vi "Main.vi"() -> ()   [LabVIEW 2013]
uses:
  <vilib>/myRIO/Common/Instrument Driver Framework/myRIO v1.0/UART/vis/myRIO v1.0 Close UART.vi
  <vilib>/myRIO/Common/Instrument Driver Framework/Utilities/vis/FPGA Ref Manager.vi
  <vilib>/myRIO/Common/Instrument Driver Framework/myRIO v1.0/myRIO v1.0 Reset FPGA.vi
  <vilib>/myRIO/Instrument Drivers/Utilities/Utilities.lvlib
panel:
  in  "Stop Button":bool
  out "logfile":path
  out "datalog record":T1
  # "Data Logger -- light+temp"
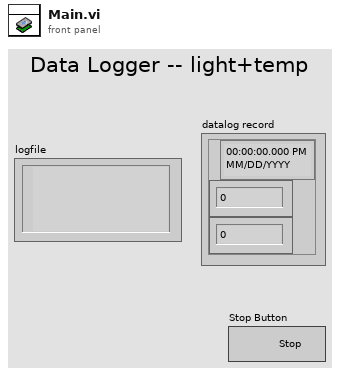
[diagram p1: front panel]
types:
  T1 = cluster{timestamp, "Numeric Control":u8, "Numeric Control":dbl}
  T2 = enum16{"open", "replace", "create", "open or create", "replace or create", "replace or create with confirmation"}
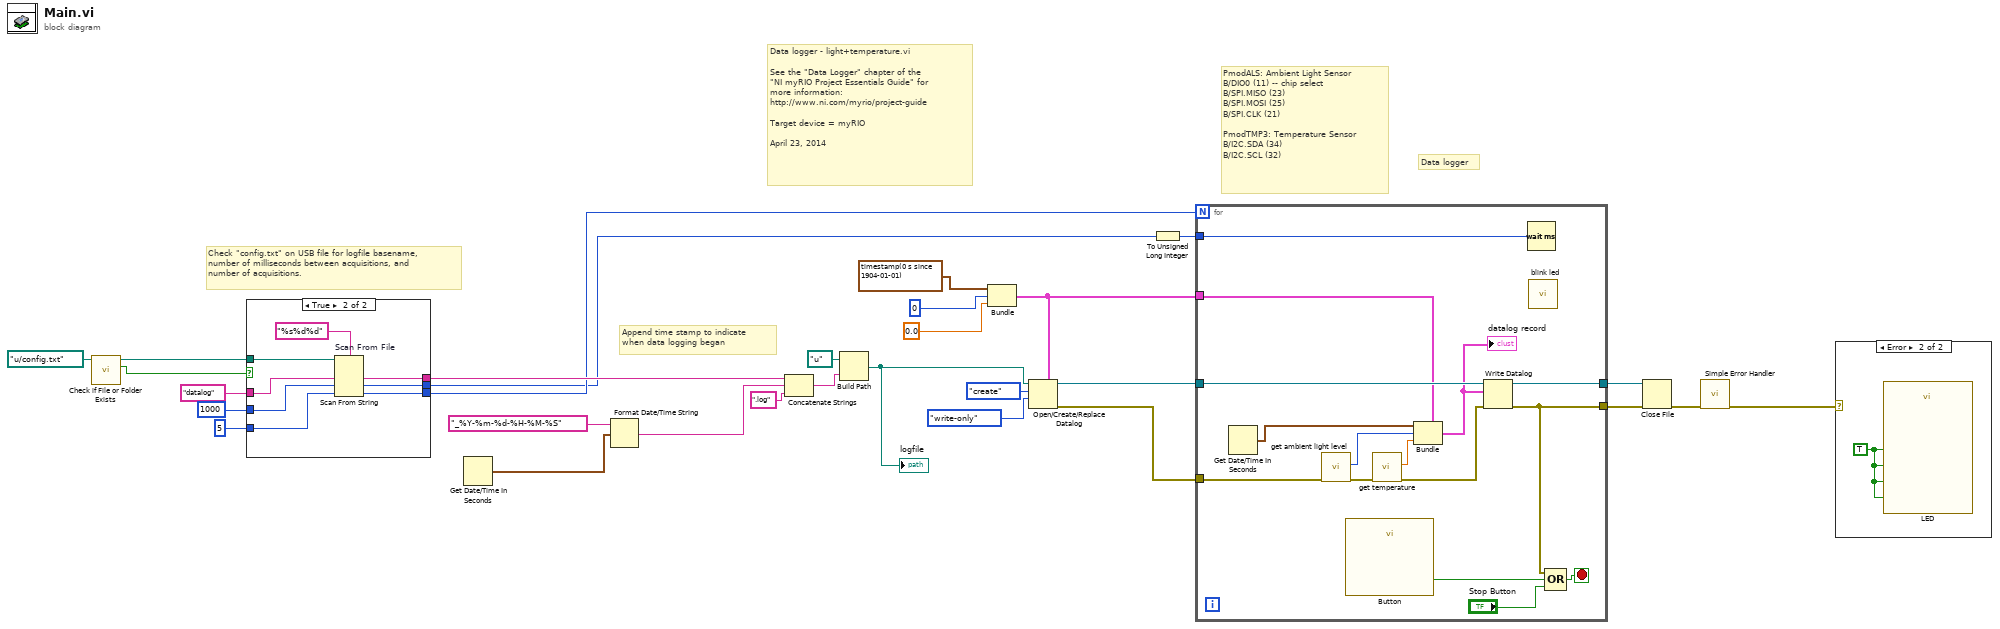
[diagram p0: block diagram]
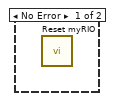
[diagram p2: hidden frame]
diagram:
  # "Data logger - light+temperature.vi\n\nSee the \"Data Logger\" chapter of the \n\"NI myRIO Project Essentials Guide\" for\nmore information: \nhttp://www.ni.com/myrio/project-guide\n\nTarget device = myRIO\n\nApril 23, 2014"
  # "Append time stamp to indicate\nwhen data logging began"
  # "Check \"config.txt\" on USB file for logfile basename,\nnumber of milliseconds between acquisitions, and\nnumber of acquisitions."
  # "Data logger"
  # "PmodALS: Ambient Light Sensor\nB/DIO0 (11) -- chip select\nB/SPI.MISO (23)\nB/SPI.MOSI (25)\nB/SPI.CLK (21)\n\nPmodTMP3: Temperature Sensor\nB/I2C.SDA (34)\nB/I2C.SCL (32)"
  n1 = call <vilib>:"Check if File or Folder Exists.vi"("path"=path "u:/config.txt") -> ("file or folder exists?"=w16:bool, "dup path"=w17:path)  [unwired: 8 in, 1 out]
  n2 = case shown="True" w16 {
    tunnel: w17 -> [_ w40]
    tunnel: [w32 w38] -> w10
    tunnel: [w31 w37] -> w2
    tunnel: [w30 w36] -> w4
    tunnel: "datalog" ("default value 1") -> [w32 w35]
    tunnel: 1000 ("default value 2") -> [w31 w34]
    tunnel: 5 ("default value 3") -> [w30 w33]
    frame False {
    }
    frame True {
      n3 = Scan From String "Scan From File"("%s%d%d" ("format string"), w40, default 1=w35, default 2=w34, default 3=w33) -> (output 1=w38:string, output 2=w37:i32, output 3=w36:i32)  [unwired: 1 in, 2 out]
    }
  }
  n4 = Get Date/Time In Seconds() -> (seconds since 1Jan1904=w12:timestamp)
  n5 = Format Date/Time String(time format string (%c)="_%Y-%m-%d-%H-%M-%S", seconds (now)=w12) -> (date/time string=w9:string)  [unwired: 1 in]
  n6 = Concatenate Strings(w10, w9, ".log" ("string")) -> (w6:string)
  n7 = Build Path(base path=path "u:/", name or relative path=w6) -> (appended path=w5:path)
  "logfile" <- w5
  n8 = Bundle(timestamp(0 s since 1904-01-01), u8 0, 0.0) -> (w23:cluster{timestamp, u8, dbl})  [unwired: 1 in]
  n9 = Open/Create/Replace Datalog(5:w23, 9:enum16{"read/write", "read-only", "write-only"}."write-only" ("access (0:read/write)"), 10:T2."create" ("operation (0:open)"), 11:w5) -> (0:w19:errorcluster, 3:w24:refnum<k1>)  [unwired: 2 in, 1 out]
  n10 = To Unsigned Long Integer(number=w2) -> (unsigned 32bit integer=w3:u32)
  n11 = for {
    N: w4 -> [_]
    tunnel: w19 -> [w55]
    tunnel: w24 -> [w54]
    tunnel: w23 -> [w53]
    tunnel: [w49] -> w22
    tunnel: [w46] -> w21
    tunnel: w3 -> [w48]
    stop <- w47 stop-if-true
    n12 = Get Date/Time In Seconds() -> (seconds since 1Jan1904=w52:timestamp)
    n13 = call "get ambient light level.vi"("error in"=w55) -> ("error out"=w45:errorcluster, "light level"=w51:u8)  [unwired: 9 in]
    n14 = call "Button"() -> ("Value"=w41:bool)  [unwired: 26 in, 1 out]
    n15 = call "get temperature.vi"("error in"=w45) -> ("error out"=w43:errorcluster, "temperature [ºC]"=w44:dbl)  [unwired: 9 in]
    n16 = Bundle(cluster=w53, w52, w51, w44) -> (w50:cluster{timestamp, u8, dbl})
    "datalog record" <- w50
    n17 = Write Datalog(4:w43, 6:w50, 7:w54) -> (0:w46:errorcluster, 3:w49:refnum<k1>)
    n18 = Wait (ms)(milliseconds to wait=w48) -> ()  [unwired: 1 out]
    n19 = call "blink led.vi"() -> ()  [unwired: 12 in]
    n20 = Compound Arithmetic op=OR(w46, w41, "Stop Button") -> (w47:bool)
  }
  n21 = Close File(refnum=w22, error in=w21) -> (error out=w20:errorcluster)  [unwired: 1 out]
  n22 = call <vilib>:"Simple Error Handler.vi"("error in (no error)"=w20) -> ("error out"=w1:errorcluster)  [unwired: 4 in, 4 out]
  n23 = case shown="Error" w1 {
    frame No Error {
      n24 = call <vilib>:"Reset myRIO.vi"() -> ()  [unwired: 11 in, 1 out]
    }
    frame Error {
      w56 = TRUE ("LED0")
      n25 = call "LED"("LED0"=w56, "LED1"=w56, "LED2"=w56, "LED3"=w56) -> ()  [unwired: 23 in, 1 out]
    }
  }
